vi "SeCrTs-RD Data reader from shared variable.vi"(0 "Config":T1, 1 "Start/Stop Log":bool[](array[boolean]), 2 "Log Name":string, 3 "C/NC":bool, 4 "Log min":dbl, 5 "error IO":errorcluster, 7 "empty?":bool) -> (19 "error out":errorcluster)   [LabVIEW 2022 SP3]
uses:
  91644d88-8a3a-46f6-9314-183f243c8ec6.vi
  3d41d14a-1e81-4e0e-8a5a-4fdd32b6dd05.vi
  Globals/SeCrTs-RD globals.vi
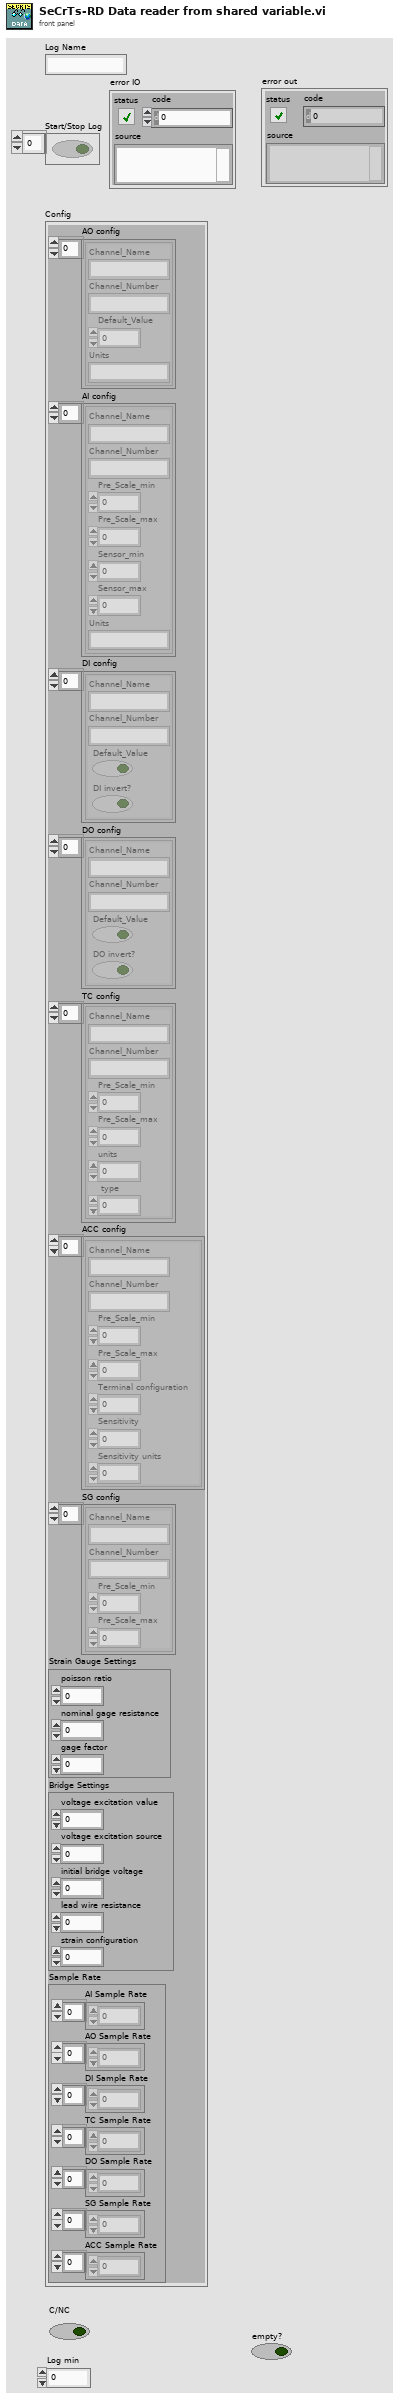
[diagram p1: front panel]
types:
  T1 = cluster{"AO config":cluster{"Channel_Name":string, "Channel_Number":string, "Default_Value":dbl, "Units":string}[], "AI config":cluster{"Channel_Name":string, "Channel_Number":string, "Pre_Scale_min":dbl, "Pre_Scale_max":dbl, "Sensor_min":dbl, "Sensor_max":dbl, "Units":string}[], "DI config":cluster{"Channel_Name":string, "Channel_Number":string, "Default_Value":bool, "DI invert?":bool}[], "DO config":cluster{"Channel_Name":string, "Channel_Number":string, "Default_Value":bool, "DO invert?":bool}[], "TC config":cluster{"Channel_Name":string, "Channel_Number":string, "Pre_Scale_min":dbl, "Pre_Scale_max":dbl, "units":i32, " type":i32}[], "ACC config":cluster{"Channel_Name":string, "Channel_Number":string, "Pre_Scale_min":dbl, "Pre_Scale_max":dbl, "Terminal configuration":i32, "Sensitivity":dbl, "Sensitivity units":i32}[], "SG config":cluster{"Channel_Name":string, "Channel_Number":string, "Pre_Scale_min":dbl, "Pre_Scale_max":dbl}[], "Strain Gauge Settings":cluster{"poisson ratio":dbl, "nominal gage resistance":dbl, "gage factor":dbl}, "Bridge Settings":cluster{"voltage excitation value":dbl, "voltage excitation source":i32, "initial bridge voltage":dbl, "lead wire resistance":dbl, "strain configuration":i32}, "Sample Rate":cluster{"AI Sample Rate":dbl[], "AO Sample Rate":dbl[], "DI Sample Rate":dbl[], "TC Sample Rate":dbl[], "DO Sample Rate":dbl[], "SG Sample Rate":dbl[], "ACC Sample Rate":dbl[]}}
  T2 = cluster{"analog names":cluster{"AI_C_Data":string[], "AI_V_Data":string[], "AO_Data":string[], "DO_Data":string[], "ACC_Data":string[], "TC Data":string[], "Drive_A_C":string[], "Drive_A_D":string[], "Drive_L_C":string[], "Drive_L_D":string[]}, "Di names":string[]}
  T3 = cluster{"AI_C_Data":string[], "AI_V_Data":string[], "AO_Data":string[], "DO_Data":string[], "ACC_Data":string[], "TC Data":string[], "Drive_A_C":string[], "Drive_A_D":string[], "Drive_L_C":string[], "Drive_L_D":string[]}
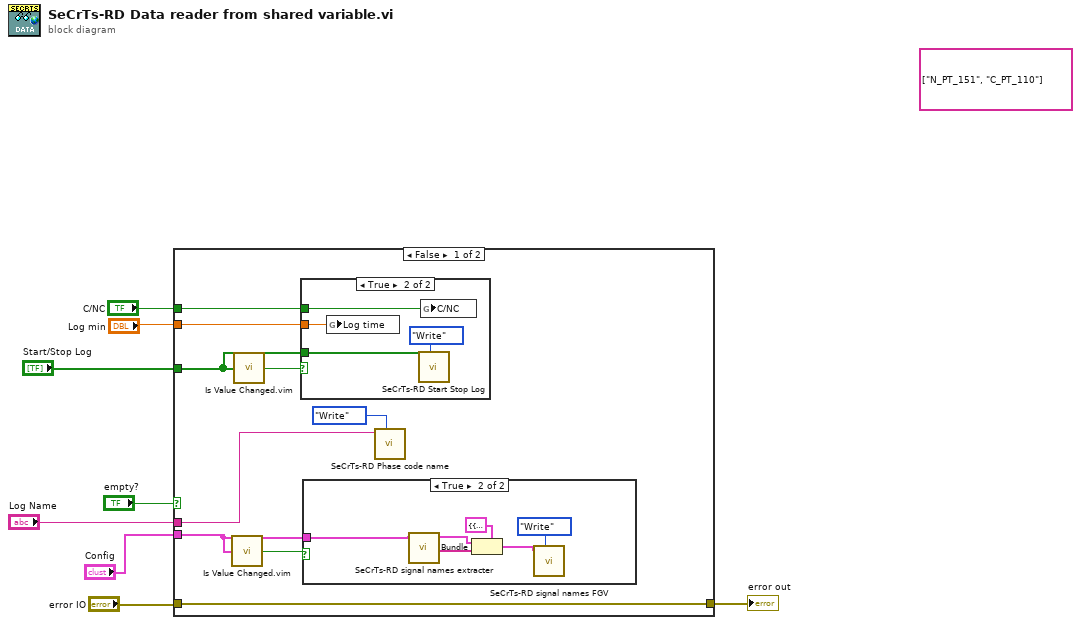
[diagram p0: block diagram]
diagram:
  (unwired) string[] ["N_PT_151", "C_PT_110"] ("element")
  n1 = case shown="False" "empty?" {
    tunnel: "Log Name" -> [w9 _]
    tunnel: "Config" -> [w15 _]
    tunnel: "Start/Stop Log" -> [w14 _]
    tunnel: "error IO" -> [w13 w28]
    tunnel: [w13 w28] -> w3
    tunnel: "C/NC" -> [w12 _]
    tunnel: "Log min" -> [w11 _]
    frame False {
      n2 = call "Is Value Changed.vim"("value"=w15) -> ("changed or first call?"=w17:bool)
      n3 = call "Is Value Changed.vim"("value"=w14) -> ("changed or first call?"=w16:bool)
      n4 = case shown="True" w16 {
        tunnel: w14 -> [_ w18]
        tunnel: w12 -> [_ w21]
        tunnel: w11 -> [_ w20]
        frame False {
        }
        frame True {
          n5 = global write "SeCrTs-RD globals.vi" "Log time"(w20) -> ()
          n6 = call "SeCrTs-RD Start Stop Log.vi"("Enum"=enum16{"Read", "Write"}."Write", "Start Stop log"=w18) -> ()  [unwired: 8 in, 2 out]
          n7 = global write "SeCrTs-RD globals.vi" "C/NC"(w21) -> ()
        }
      }
      n8 = case shown="True" w17 {
        tunnel: w15 -> [_ w22]
        frame False {
        }
        frame True {
          n9 = call "SeCrTs-RD signal names extracter.vi"("input cluster"=w22) -> ("Di names"=w26:string[], "analog names"=w25:T3)  [unwired: 9 in]
          n10 = Bundle(cluster=T2 {"analog names"={"AI_C_Data"=[], "AI_V_Data"=[], "AO_Data"=[], "DO_Data"=[], "ACC_Data"=[], "TC Data"=[], "Drive_A_C"=[], "Drive_A_D"=[], "Drive_L_C"=[], "Drive_L_D"=[]}, "Di names"=[]}, "analog names"=w25, "Di names"=w26) -> (w27:T2)
          n11 = call "SeCrTs-RD signal names FGV.vi"("Enum"=enum16{"Read", "Write"}."Write", "Signal names"=w27) -> ()  [unwired: 8 in, 2 out]
        }
      }
      n12 = call "SeCrTs-RD Phase code name.vi"("Enum"=enum16{"Read", "Write"}."Write", "Phase code W"=w9) -> ()  [unwired: 8 in, 2 out]
    }
    frame True {
    }
  }
  "error out" <- w3
